vi "Read (All Parameters).vi"(7 "Timeout (10000 ms)":u32=10000, 8 "error in (no error)":errorcluster, 11 "VISA resource name":refnum<visa-resource-name>) -> (0 "error out":errorcluster, 2 "Parameter Values":T1, 3 "VISA resource name out":refnum<visa-resource-name>)   [LabVIEW 2012, in "Stanford Research 830.lvlib"]
doc: "Reads all the available parameters from the instrument.\n\n<B>Note:</B>\n\nThis VI only reads multiple parameters, not multiple points of the same parameter."
uses:
  <instrlib>/Stanford Research 830/Stanford Research 830.lvlib
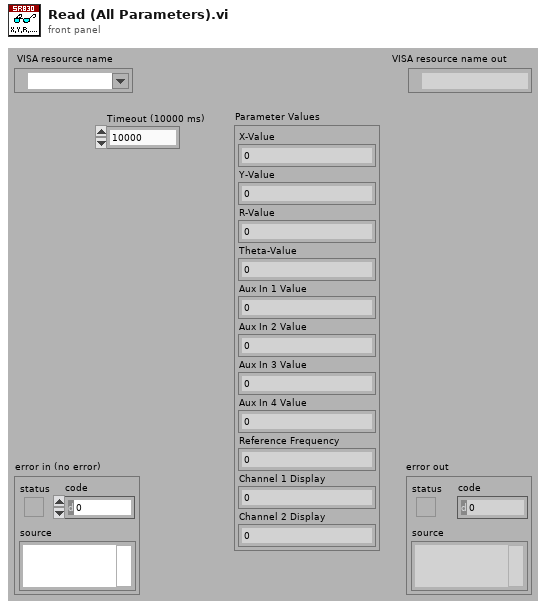
[diagram p1: front panel]
types:
  T1 = cluster{"X-Value":dbl, "Y-Value":dbl, "R-Value":dbl, "Theta-Value":dbl, "Aux In 1 Value":dbl, "Aux In 2 Value":dbl, "Aux In 3 Value":dbl, "Aux In 4 Value":dbl, "Reference Frequency":dbl, "Channel 1 Display":dbl, "Channel 2 Display":dbl}
  T2 = cluster{dbl, dbl, dbl, dbl, dbl, dbl, dbl, dbl, dbl, dbl, dbl}
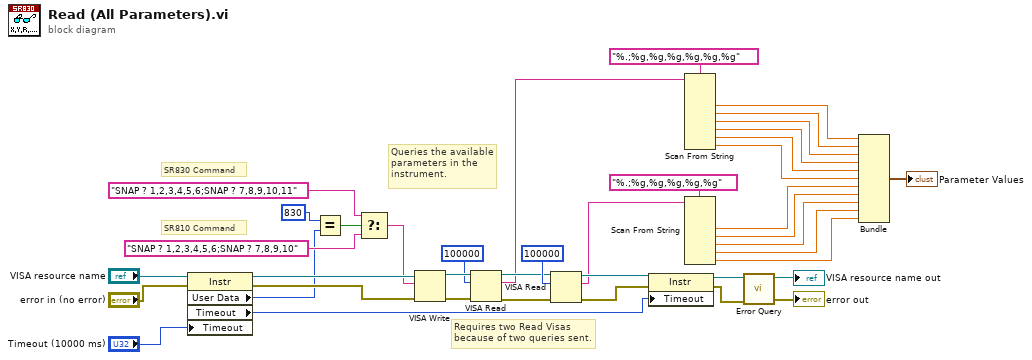
[diagram p0: block diagram]
diagram:
  # "SR810 Command"
  # "SR830 Command"
  # "Requires two Read Visas because of two queries sent."
  # "Queries the available parameters in the instrument."
  n1 = property class="Instr"(reference="VISA resource name", error in="error in (no error)", "Timeout"="Timeout (10000 ms)") -> (reference out=w38:refnum<visa-resource-name>, error out=w37:errorcluster, "User Data"=w1:u32, "Timeout"=w8:u32)
  n2 = Equal?(x=u32 830, y=w1) -> (x = y?=w3:bool)
  n3 = Select(t="SNAP ? 1,2,3,4,5,6;SNAP ? 7,8,9,10,11" ("write buffer"), s=w3, f="SNAP ? 1,2,3,4,5,6;SNAP ? 7,8,9,10" ("write buffer")) -> (s? t:f=w4:string)
  n4 = VISA Write(VISA resource name=w38, write buffer=w4, error in (no error)=w37) -> (VISA resource name out=w39:refnum<visa-resource-name>, error out=w40:errorcluster)  [unwired: 1 out]
  n5 = VISA Read(VISA resource name=w39, byte count=u32 100000, error in (no error)=w40) -> (VISA resource name out=w22:refnum<visa-resource-name>, read buffer=w17:string, error out=w21:errorcluster)  [unwired: 1 out]
  n6 = VISA Read(VISA resource name=w22, byte count=u32 100000, error in (no error)=w21) -> (VISA resource name out=w20:refnum<visa-resource-name>, read buffer=w16:string, error out=w19:errorcluster)  [unwired: 1 out]
  n7 = property class="Instr"(reference=w20, error in=w19, "Timeout"=w8) -> (reference out=w32:refnum<visa-resource-name>, error out=w33:errorcluster)
  n8 = Scan From String(format string="%.;%g,%g,%g,%g,%g,%g", input string=w17) -> (output 1=w28:dbl, output 2=w27:dbl, output 3=w26:dbl, output 4=w25:dbl, output 5=w24:dbl, output 6=w18:dbl)  [unwired: 8 in, 3 out]
  n9 = Scan From String(format string="%.;%g,%g,%g,%g,%g", input string=w16) -> (output 1=w15:dbl, output 2=w14:dbl, output 3=w13:dbl, output 4=w12:dbl, output 5=w11:dbl)  [unwired: 7 in, 3 out]
  n10 = call <instrlib>:"Error Query.vi"("error in (no error)"=w33, "VISA resource name"=w32) -> ("error out"=→"error out":errorcluster, "VISA resource name out"=→"VISA resource name out":refnum<visa-resource-name>)  [unwired: 7 in, 1 out]
  n11 = Bundle(w28, w27, w26, w25, w24, w18, w15, w14, w13, w12, w11) -> (→"Parameter Values":T2)  [unwired: 1 in]
